vi "Solenoids.vi"(8 "error in":errorcluster) -> (0 "error out":errorcluster, 1 "error out 2":errorcluster)   [LabVIEW 2013]
uses:
  <vilib>/Rock Robotics/WPI/Solenoid/WPI_SolenoidValue.ctl
  SorD_Solenoid.ctl
  <vilib>/Rock Robotics/SystemInterfaces/Typedef/FPGA_TypedefSolenoidModule.ctl
  <vilib>/Rock Robotics/WPI/Solenoid/WPI_SolenoidChannel.ctl
  <vilib>/Rock Robotics/WPI/Solenoid/WPI_SolenoidOpenSingle.vi
  <vilib>/Rock Robotics/WPI/Solenoid/WPI_SolenoidSetEnum.vi
  <vilib>/Rock Robotics/WPI/Solenoid/WPI_SolenoidOpenDouble.vi
panel:
  in  "Single or Double Solenoid":T1
  in  "DoubleTwo":T2
  in  "DoubleOne":T2
  in  "Solenoid4":T2
  in  "Solenoid3":T2
  in  "Solenoid2":T2
  in  "Solenoid1":T2
  # "Single"
  # "Double"
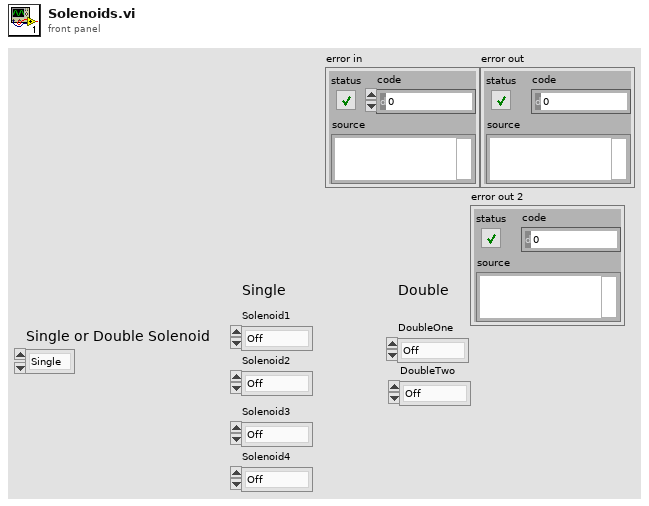
[diagram p1: front panel]
types:
  T1 = typedef "SorD_Solenoid.ctl" = enum16{"Single", "Double"}
  T2 = typedef "WPI_SolenoidValue.ctl" = enum16{"Off", "On", "Forward", "Reverse"}
  T3 = typedef "WPI_SolenoidChannel.ctl" = enum8{"Solenoid 1", "Solenoid 2", "Solenoid 3", "Solenoid 4", "Solenoid 5", "Solenoid 6", "Solenoid 7", "Solenoid 8", "Invalid"}
  T4 = typedef "FPGA_TypedefSolenoidModule.ctl" = enum16{"Solenoid Module 1", "Solenoid Module 2"}
  T5 = typedef "WPI_SolenoidDevRef.ctl" = cluster{"DevStatus":errorcluster, "Solenoid Module":T4, "Forward Solenoid Channel":T3, "Reverse Solenoid Channel":T3}
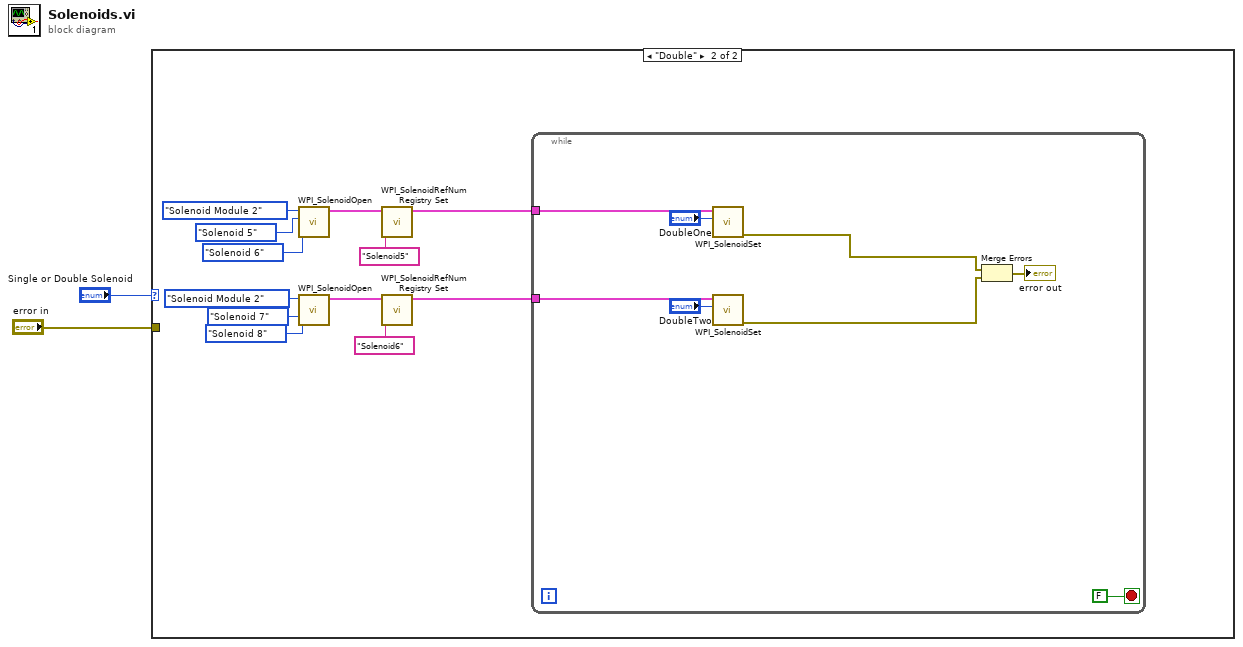
[diagram p0: block diagram]
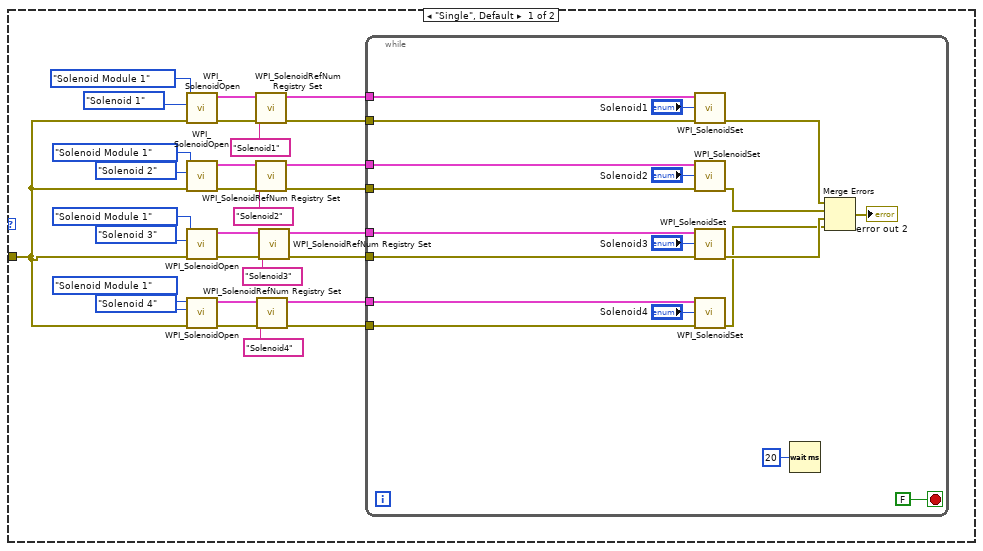
[diagram p2: hidden frame]
diagram:
  n1 = case shown="\"Double\"" "Single or Double Solenoid" {
    tunnel: "error in" -> [w11 _]
    frame "Single", Default {
      n2 = call-poly <vilib>:"WPI_SolenoidOpen.vi"("error in (no error)"=w11, "Solenoid Channel"=WPI_SolenoidChannel."Solenoid 1", "Solenoid Module (Module 1)"=FPGA_TypedefSolenoidModule."Solenoid Module 1") -> ("error out"=w10:errorcluster, "SolenoidDevRef"=w19:T5)  [unwired: 7 in]
      n3 = call-poly <vilib>:"WPI_SolenoidOpen.vi"("error in (no error)"=w11, "Solenoid Channel"=WPI_SolenoidChannel."Solenoid 2", "Solenoid Module (Module 1)"=FPGA_TypedefSolenoidModule."Solenoid Module 1") -> ("error out"=w8:errorcluster, "SolenoidDevRef"=w18:T5)  [unwired: 7 in]
      n4 = call-poly <vilib>:"WPI_SolenoidOpen.vi"("error in (no error)"=w11, "Solenoid Channel"=WPI_SolenoidChannel."Solenoid 3", "Solenoid Module (Module 1)"=FPGA_TypedefSolenoidModule."Solenoid Module 1") -> ("error out"=w6:errorcluster, "SolenoidDevRef"=w17:T5)  [unwired: 7 in]
      n5 = call-poly <vilib>:"WPI_SolenoidOpen.vi"("error in (no error)"=w11, "Solenoid Channel"=WPI_SolenoidChannel."Solenoid 4", "Solenoid Module (Module 1)"=FPGA_TypedefSolenoidModule."Solenoid Module 1") -> ("error out"=w4:errorcluster, "SolenoidDevRef"=w16:T5)  [unwired: 7 in]
      n6 = call <vilib>:"WPI_SolenoidRefNum Registry Set.vi"("error in (no error)"=w10, "refnum name"="Solenoid1", "SolenoidDevRef"=w19) -> ("error out"=w9:errorcluster, "SolenoidDevRef"=w15:T5)  [unwired: 7 in]
      n7 = call <vilib>:"WPI_SolenoidRefNum Registry Set.vi"("error in (no error)"=w8, "refnum name"="Solenoid2", "SolenoidDevRef"=w18) -> ("error out"=w7:errorcluster, "SolenoidDevRef"=w14:T5)  [unwired: 7 in]
      n8 = call <vilib>:"WPI_SolenoidRefNum Registry Set.vi"("error in (no error)"=w4, "refnum name"="Solenoid4", "SolenoidDevRef"=w16) -> ("error out"=w3:errorcluster, "SolenoidDevRef"=w12:T5)  [unwired: 7 in]
      n9 = call <vilib>:"WPI_SolenoidRefNum Registry Set.vi"("error in (no error)"=w6, "refnum name"="Solenoid3", "SolenoidDevRef"=w17) -> ("error out"=w5:errorcluster, "SolenoidDevRef"=w13:T5)  [unwired: 7 in]
      n10 = while {
        tunnel: w15 -> [w49]
        tunnel: w14 -> [w48]
        tunnel: w13 -> [w47]
        tunnel: w12 -> [w46]
        tunnel: w9 -> [w41]
        tunnel: w7 -> [w40]
        tunnel: w5 -> [w39]
        tunnel: w3 -> [w38]
        stop <- FALSE stop-if-true
        n11 = call-poly <vilib>:"WPI_SolenoidSet.vi"("error in (no error)"=w41, "Value"="Solenoid1", "SolenoidDevRef"=w49) -> ("error out"=w37:errorcluster)  [unwired: 7 in, 1 out]
        n12 = call-poly <vilib>:"WPI_SolenoidSet.vi"("error in (no error)"=w40, "Value"="Solenoid2", "SolenoidDevRef"=w48) -> ("error out"=w36:errorcluster)  [unwired: 7 in, 1 out]
        n13 = call-poly <vilib>:"WPI_SolenoidSet.vi"("error in (no error)"=w39, "Value"="Solenoid3", "SolenoidDevRef"=w47) -> ("error out"=w35:errorcluster)  [unwired: 7 in, 1 out]
        n14 = call-poly <vilib>:"WPI_SolenoidSet.vi"("error in (no error)"=w38, "Value"="Solenoid4", "SolenoidDevRef"=w46) -> ("error out"=w34:errorcluster)  [unwired: 7 in, 1 out]
        n15 = Wait (ms)(milliseconds to wait=u32 20) -> ()  [unwired: 1 out]
        n16 = Merge Errors(w37, w36, w35, w34) -> (→"error out 2":errorcluster)
      }
    }
    frame "Double" {
      n17 = call-poly <vilib>:"WPI_SolenoidOpen.vi"("Reverse Solenoid Channel"=WPI_SolenoidChannel."Solenoid 6", "Forward Solenoid Channel"=WPI_SolenoidChannel."Solenoid 5" ("Solenoid Channel"), "Solenoid Module (Module 1)"=FPGA_TypedefSolenoidModule."Solenoid Module 2") -> ("SolenoidDevRef"=w58:T5)  [unwired: 7 in, 1 out]
      n18 = call-poly <vilib>:"WPI_SolenoidOpen.vi"("Reverse Solenoid Channel"=WPI_SolenoidChannel."Solenoid 8", "Forward Solenoid Channel"=WPI_SolenoidChannel."Solenoid 7" ("Solenoid Channel"), "Solenoid Module (Module 1)"=FPGA_TypedefSolenoidModule."Solenoid Module 2") -> ("SolenoidDevRef"=w57:T5)  [unwired: 7 in, 1 out]
      n19 = call <vilib>:"WPI_SolenoidRefNum Registry Set.vi"("refnum name"="Solenoid5", "SolenoidDevRef"=w58) -> ("SolenoidDevRef"=w53:T5)  [unwired: 8 in, 1 out]
      n20 = call <vilib>:"WPI_SolenoidRefNum Registry Set.vi"("refnum name"="Solenoid6", "SolenoidDevRef"=w57) -> ("SolenoidDevRef"=w54:T5)  [unwired: 8 in, 1 out]
      n21 = while {
        tunnel: w54 -> [w69]
        tunnel: w53 -> [w68]
        stop <- FALSE stop-if-true
        n22 = call-poly <vilib>:"WPI_SolenoidSet.vi"("Value"="DoubleOne", "SolenoidDevRef"=w68) -> ("error out"=w65:errorcluster)  [unwired: 8 in, 1 out]
        n23 = call-poly <vilib>:"WPI_SolenoidSet.vi"("Value"="DoubleTwo", "SolenoidDevRef"=w69) -> ("error out"=w64:errorcluster)  [unwired: 8 in, 1 out]
        n24 = Merge Errors(w65, w64) -> (→"error out":errorcluster)
      }
    }
  }
